vi "VIPropertyPicker.vi"() -> ()   [LabVIEW 2019]
uses:
  VIPropertyPicker/VIPropertyPicker.lvlib
  lib/UI/TreeControl/TreeControlLib.lvlib
  ae6c83ba-cc00-42a4-a275-f8b2c398fdcb.vi
panel:
  out "Last Selection":string
  out "UserMenuNames":string[](array[string])
  out "UserMenuTags":string[](array[string])
  in  "Reload1":bool caption="Reload (CTRL+R)"
  in  "VI Properties":string[](tree)
  in  "Reload2":bool caption="Reload (Ctrl+R)"
  in  "VI List":string(tree)
  in  "Script":string
  in  "Append to Editor in ScriptManager":bool
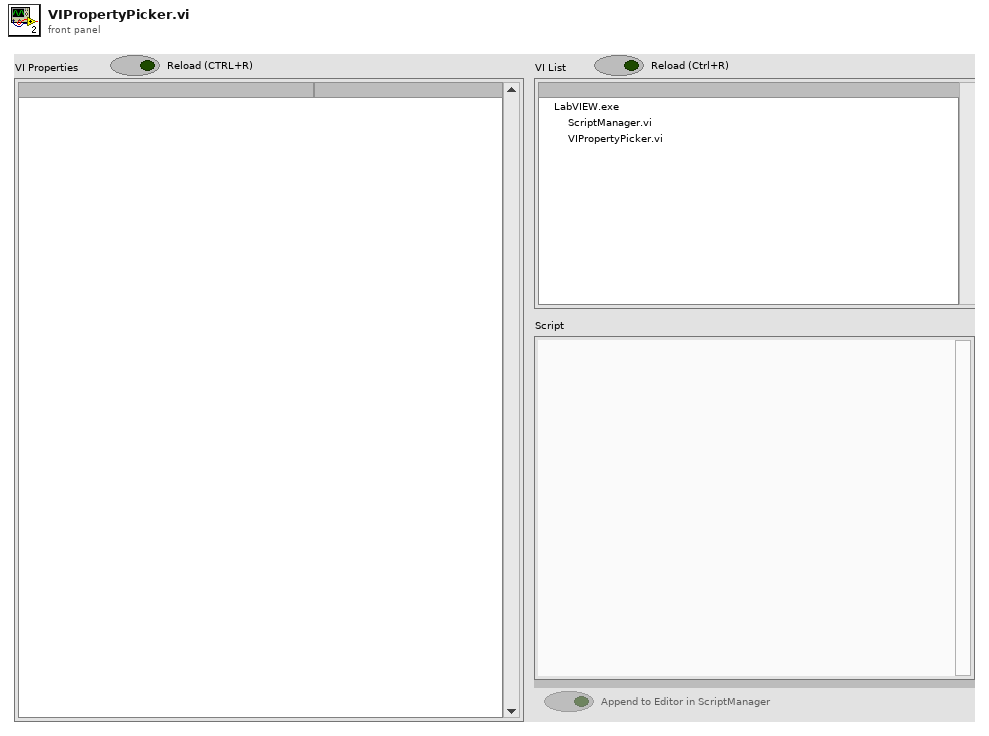
[diagram p1: front panel]
types:
  T1 = enum8{"Enabled", "Disabled", "Disabled and Grayed Out"}
  T2 = cluster{"Name":string, "Include Shift Key?":bool, "Include Ctrl Key?":bool, "Shortcut Key":string}[]
  T3 = cluster{"Closed Nodes":string[], "Selection":string[], "Defer Panel Update":bool, "FocusItem":string}
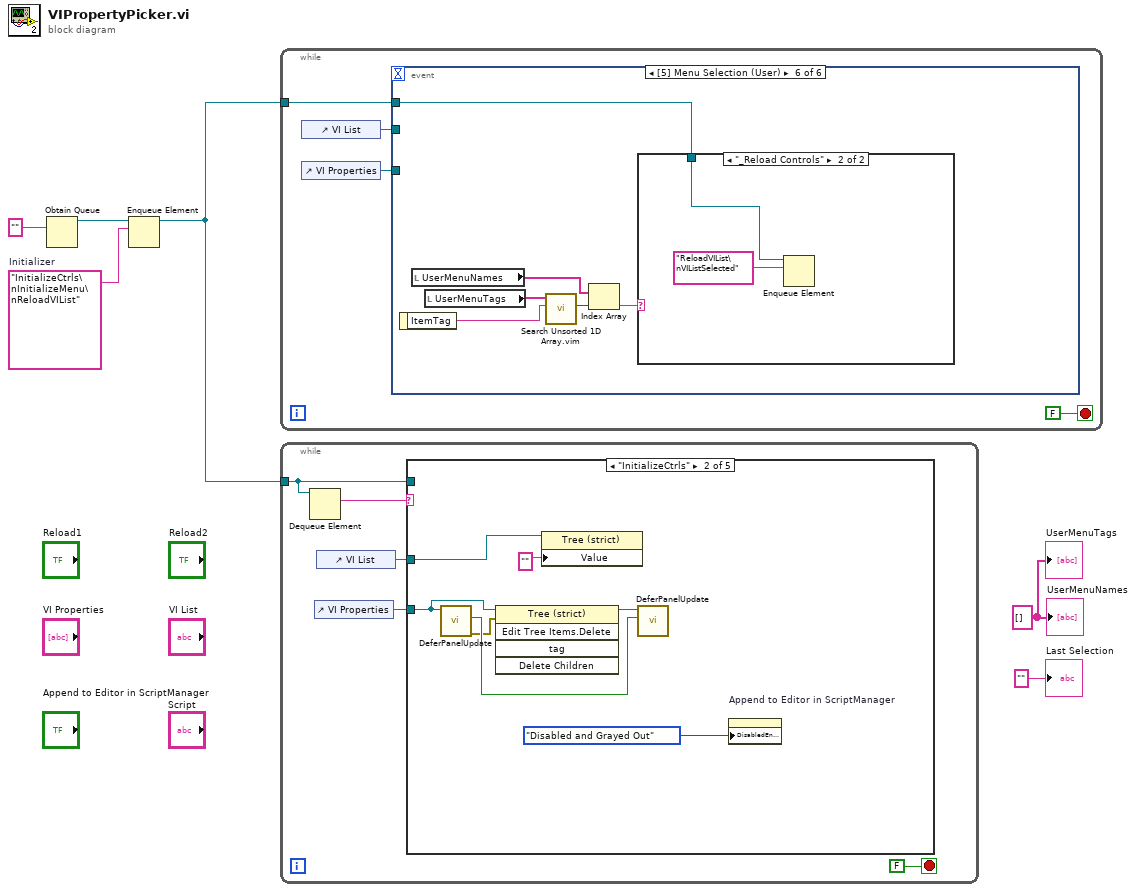
[diagram p0: block diagram]
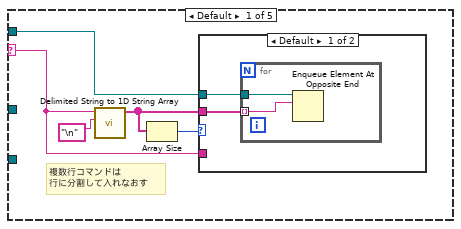
[diagram p2: hidden frame]
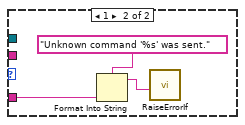
[diagram p3: hidden frame]
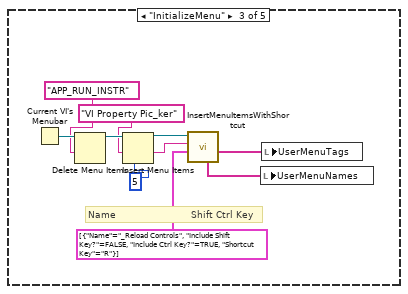
[diagram p4: hidden frame]
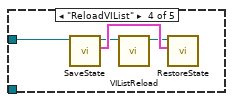
[diagram p5: hidden frame]
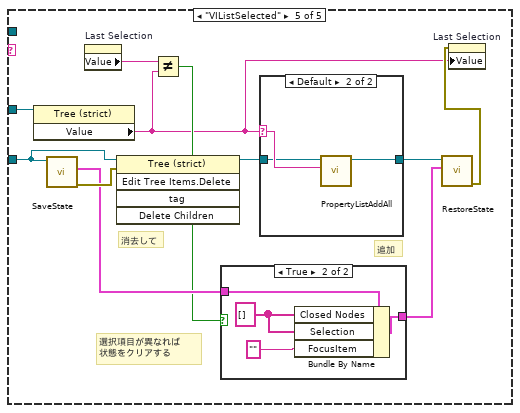
[diagram p6: hidden frame]
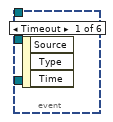
[diagram p9: hidden frame]
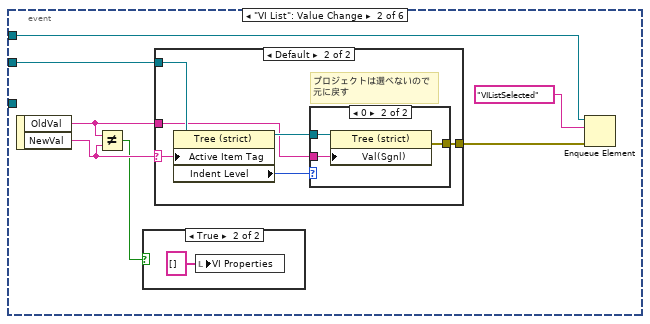
[diagram p10: hidden frame]
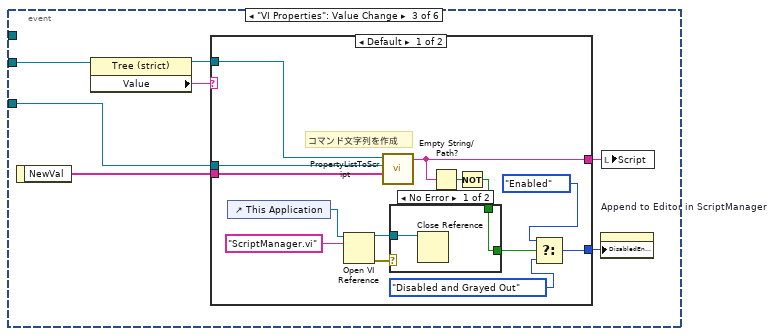
[diagram p14: hidden frame]
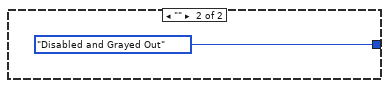
[diagram p16: hidden frame]
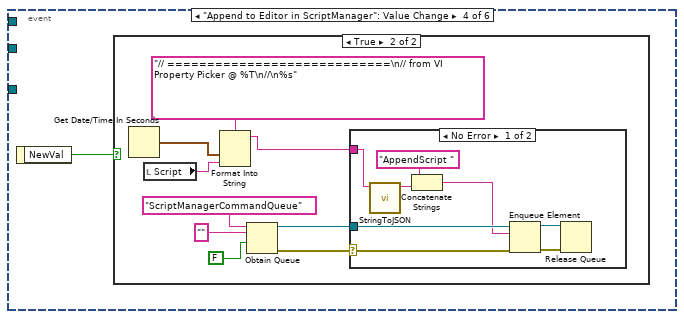
[diagram p17: hidden frame]
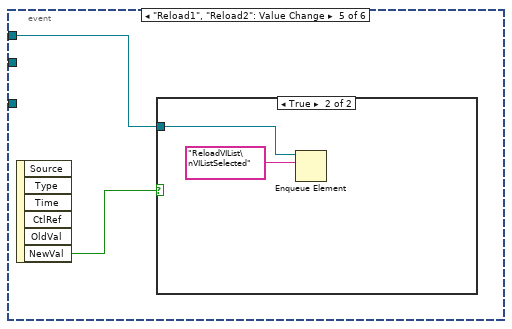
[diagram p20: hidden frame]
diagram:
  w1 = string[] [] ("UserMenuNames")
  w3 = "InitializeCtrls\nInitializeMenu\nReloadVIList"  # Initializer
  n1 = Obtain Queue(element data type="") -> (queue out=w5:refnum<queue>)  [unwired: 4 in, 2 out]
  n2 = Enqueue Element(queue=w5, element=w3) -> (queue out=w4:refnum<queue>)  [unwired: 2 in, 2 out]
  n3 = while {
    tunnel: w4 -> [w9]
    stop <- FALSE stop-if-true
    n4 = control-ref of="VI List"() -> (w8:refnum<vi>)
    n5 = control-ref of="VI Properties"() -> (w7:refnum<vi>)
    n6 = event shown="[5] Menu Selection (User)" {
      selector: _ -> [_ _ _ _ _ _]
      dyn-events: _ -> [_ _ _ _ _ _]
      timeout: _ -> [_ _ _ _ _ _]
      tunnel: w9 -> [_ w16 _ _ w70 w74]
      tunnel: w8 -> [_ w17 w31 _ _ _]
      tunnel: w7 -> [_ _ w33 _ _ _]
      event Timeout {
        n7 = event-data() -> ()  [unwired: 1 in, 3 out]
      }
      event "VI List": Value Change {
        n8 = event-data() -> ("OldVal"=w13:string, "NewVal"=w12:string)  [unwired: 1 in]
        n9 = Not Equal?(x=w13, y=w12) -> (x != y?=w11:bool)
        n10 = case shown="True" w11 {
          frame False {
          }
          frame True {
            n11 = local write "VI Properties"(string[] [] ("VI Properties")) -> ()
          }
        }
        n12 = case shown="Default" w12 {
          selector: w12 -> [_ w19]
          tunnel: w17 -> [_ w24]
          tunnel: [_ w21] -> w14
          tunnel: w13 -> [_ w20]
          frame "" {
          }
          frame Default {
            # "プロジェクトは選べないので\n元に戻す"
            n13 = property class="Tree (strict)"(reference=w24, "Active Item Tag"=w19) -> (reference out=w23:refnum<vi>, "Indent Level"=w22:i32)  [unwired: 1 in, 1 out]
            n14 = case shown="0" w22 {
              tunnel: w23 -> [_ w27]
              tunnel: w20 -> [_ w26]
              tunnel: [_ w25] -> w21
              frame Default {
              }
              frame 0 {
                n15 = property class="Tree (strict)"(reference=w27, "Val(Sgnl)"=w26) -> (error out=w25:errorcluster)  [unwired: 1 in, 1 out]
              }
            }
          }
        }
        n16 = Enqueue Element(queue=w16, element="VIListSelected", error in (no error)=w14) -> ()  [unwired: 1 in, 3 out]
      }
      event "VI Properties": Value Change {
        n17 = event-data() -> ("NewVal"=w34:string[])  [unwired: 1 in]
        n18 = property class="Tree (strict)"(reference=w31) -> (reference out=w29:refnum<vi>, "Value"=w30:string)  [unwired: 1 in, 1 out]
        n19 = case shown="Default" w30 {
          tunnel: w34 -> [w48 _]
          tunnel: w33 -> [w47 _]
          tunnel: [w42 _] -> w32
          tunnel: w29 -> [w35 _]
          tunnel: [w36 T1."Disabled and Grayed Out" ("Disabled")] -> w28
          frame Default {
            # "コマンド文字列を作成"
            n20 = control-ref of="This Application"() -> (w46:refnum<vi>)
            n21 = Open VI Reference(application reference (local)=w46, vi path="ScriptManager.vi") -> (vi reference=w44:refnum<vi>, error out=w43:errorcluster)  [unwired: 4 in]
            n22 = call "PropertyListToScript.vi"("NewVal"=w48, "VI Properties"=w47, "TreeControl in"=w35) -> ("Script"=w42:string)  [unwired: 8 in]
            n23 = Empty String/Path?(string/path=w42) -> (empty?=w41:bool)
            n24 = Not(x=w41) -> (.not. x?=w39:bool)
            n25 = case shown="No Error" w43 {
              tunnel: w44 -> [w50 _]
              tunnel: [w49 _] -> w38
              tunnel: w39 -> [w49 _]
              frame No Error {
                n26 = Close Reference(reference=w50) -> ()  [unwired: 1 in, 1 out]
              }
              frame Error {
              }
            }
            n27 = Select(t=T1."Enabled" ("Disabled"), s=w38, f=T1."Disabled and Grayed Out" ("Disabled")) -> (s? t:f=w36:T1)
          }
          frame "" {
          }
        }
        n28 = property on="Append to Editor in ScriptManager" class="Bool (strict)"("DisabledEnum"=w28) -> ()  [unwired: 2 in, 2 out]
        n29 = local write "Script"(w32) -> ()
      }
      event "Append to Editor in ScriptManager": Value Change {
        n30 = event-data() -> ("NewVal"=w52:bool)  [unwired: 1 in]
        n31 = case shown="True" w52 {
          frame False {
          }
          frame True {
            n32 = Get Date/Time In Seconds() -> (seconds since 1Jan1904=w53:timestamp)
            n33 = local read "Script"() -> (w54:string)
            n34 = Format Into String(format string="// ============================\n// from VI Property Picker @ %T\n//\n%s", w53, w54) -> (resulting string=w56:string)  [unwired: 2 in, 1 out]
            n35 = Obtain Queue(name (unnamed)="ScriptManagerCommandQueue", element data type="", create if not found? (T)=FALSE) -> (queue out=w58:refnum<queue>, error out=w57:errorcluster)  [unwired: 2 in, 1 out]
            n36 = case shown="No Error" w57 {
              selector: w57 -> [w62 _]
              tunnel: w56 -> [w69 _]
              tunnel: w58 -> [w67 _]
              frame No Error {
                n37 = call "StringToJSON.vi"("input text"=w69) -> ("JSON string"=w68:string)  [unwired: 10 in]
                n38 = Concatenate Strings("AppendScript " ("string"), w68) -> (w64:string)
                n39 = Enqueue Element(queue=w67, element=w64, error in (no error)=w62) -> (queue out=w66:refnum<queue>, error out=w65:errorcluster)  [unwired: 1 in, 1 out]
                n40 = Release Queue(queue=w66, error in (no error)=w65) -> ()  [unwired: 1 in, 3 out]
              }
              frame Error {
              }
            }
          }
        }
      }
      event "Reload1", "Reload2": Value Change {
        n41 = event-data() -> ("NewVal"=w71:bool)  [unwired: 1 in, 5 out]
        n42 = case shown="True" w71 {
          tunnel: w70 -> [_ w73]
          frame False {
          }
          frame True {
            n43 = Enqueue Element(queue=w73, element="ReloadVIList\nVIListSelected") -> ()  [unwired: 2 in, 3 out]
          }
        }
      }
      event Menu Selection (User) {
        n44 = event-data() -> ("ItemTag"=w78:string)  [unwired: 1 in]
        n45 = local read "UserMenuNames"() -> (w77:string[])
        n46 = local read "UserMenuTags"() -> (w79:string[])
        n47 = call "Search Unsorted 1D Array.vim"("element"=w78, "unsorted 1D array"=w79) -> ("index of element"=w76:i32)  [unwired: 9 in]
        n48 = Index Array(array=w77, index=w76) -> (element=w75:string)
        n49 = case shown="\"_Reload Controls\"" w75 {
          selector: w75 -> [w80 _]
          tunnel: w74 -> [_ w83]
          frame Default {
            n50 = Concatenate Strings("Unknown menu item was selected:\n", w80) -> (w82:string)
            n51 = call "RaiseErrorIf.vi"("error message"=w82) -> ()  [unwired: 10 in, 1 out]
          }
          frame "_Reload Controls" {
            n52 = Enqueue Element(queue=w83, element="ReloadVIList\nVIListSelected") -> ()  [unwired: 2 in, 3 out]
          }
        }
      }
    }
  }
  n53 = while {
    tunnel: w4 -> [w86]
    stop <- FALSE stop-if-true
    n54 = Dequeue Element(queue=w86) -> (element=w88:string)  [unwired: 2 in, 3 out]
    n55 = control-ref of="VI Properties"() -> (w85:refnum<vi>)
    n56 = control-ref of="VI List"() -> (w87:refnum<vi>)
    n57 = case shown="\"InitializeCtrls\"" w88 {
      selector: w88 -> [w92 _ _ _ _]
      tunnel: w87 -> [_ w104 _ w119 w133]
      tunnel: w86 -> [w90 _ _ _ _]
      tunnel: w85 -> [_ w106 _ _ w130]
      frame Default {
        # "複数行コマンドは\n行に分割して入れなおす"
        n58 = call <vilib>:"Delimited String to 1D String Array.vi"("delimiter"="\n", "delimited string"=w92) -> ("string array"=w91:string[])  [unwired: 9 in]
        n59 = Array Size(array=w91) -> (size(s)=w93:i32)
        n60 = case shown="Default" w93 {
          tunnel: w92 -> [_ w100]
          tunnel: w91 -> [w96 _]
          tunnel: w90 -> [w95 _]
          frame Default {
            n61 = for {
              tunnel: w96 -> [w97] mode=indexing
              tunnel: w95 -> [w98]
              n62 = Enqueue Element At Opposite End(queue=w98, element=w97) -> ()  [unwired: 2 in, 3 out]
            }
          }
          frame 1 {
            n63 = Format Into String(format string="Unknown command '%s' was sent." ("error message"), w100) -> (resulting string=w99:string)  [unwired: 2 in, 1 out]
            n64 = call "RaiseErrorIf.vi"("error message"=w99) -> ()  [unwired: 10 in, 1 out]
          }
        }
      }
      frame "InitializeCtrls" {
        n65 = call "DeferPanelUpdate.vi"("Control in"=w106) -> ("error out"=w107:errorcluster, "Defer Panel Updates Old"=w108:bool)  [unwired: 8 in, 1 out]
        n66 = invoke class="Tree (strict)" method="Edit Tree Items.Delete"(reference=w106, error in=w107) -> (reference out=w105:refnum<vi>)  [unwired: 3 in, 4 out]
        n67 = property class="Tree (strict)"(reference=w104, "Value"="") -> ()  [unwired: 1 in, 2 out]
        n68 = call "DeferPanelUpdate.vi"("Defer Panel Updates (T)"=w108, "Control in"=w105) -> ()  [unwired: 7 in, 3 out]
        n69 = property on="Append to Editor in ScriptManager" class="Bool (strict)"("DisabledEnum"=T1."Disabled and Grayed Out" ("Disabled")) -> ()  [unwired: 2 in, 2 out]
      }
      frame "InitializeMenu" {
        # "Name                         Shift Ctrl Key"
        n70 = Current VI's Menubar() -> (w115:refnum<k9>)
        n71 = Delete Menu Items(7:"APP_RUN_INSTR", 9:w115) -> (3:w118:refnum<k9>)  [unwired: 2 in, 1 out]
        n72 = Insert Menu Items(4:5, 7:"VI Property Pic_ker", 9:w118) -> (1:w117:string, 3:w116:refnum<k9>)  [unwired: 3 in, 1 out]
        n73 = call "InsertMenuItemsWithShortcut.vi"("Sub Items"=T2 [{"Name"="_Reload Controls", "Include Shift Key?"=FALSE, "Include Ctrl Key?"=TRUE, "Shortcut Key"="R"}] ("Menu Short Cut"), "Target Tag"=w117, "menu ref"=w116) -> ("Sub Item Tags"=w110:string[], "Sub Item Names"=w109:string[])  [unwired: 5 in, 2 out]
        n74 = local write "UserMenuNames"(w109) -> ()
        n75 = local write "UserMenuTags"(w110) -> ()
      }
      frame "ReloadVIList" {
        n76 = call "SaveState.vi"("TreeControl in"=w119) -> ("State"=w122:T3, "TreeControl out"=w120:refnum<vi>)  [unwired: 8 in, 1 out]
        n77 = call "VIListReload.vi"("VI List in"=w120) -> ("VI List out"=w121:refnum<vi>)  [unwired: 10 in]
        n78 = call "RestoreState.vi"("State"=w122, "TreeControl in"=w121) -> ()  [unwired: 8 in, 2 out]
      }
      frame "VIListSelected" {
        # "選択項目が異なれば\n状態をクリアする"
        # "追加"
        # "消去して"
        n79 = property class="Tree (strict)"(reference=w133) -> ("Value"=w123:string)  [unwired: 1 in, 2 out]
        n80 = call "SaveState.vi"("TreeControl in"=w130) -> ("error out"=w129:errorcluster, "State"=w127:T3)  [unwired: 8 in, 1 out]
        n81 = property on="Last Selection" class="Str"() -> ("Value"=w128:string)  [unwired: 2 in, 2 out]
        n82 = invoke class="Tree (strict)" method="Edit Tree Items.Delete"(reference=w130, error in=w129) -> (reference out=w132:refnum<vi>)  [unwired: 3 in, 4 out]
        n83 = Not Equal?(x=w128, y=w123) -> (x != y?=w125:bool)
        n84 = case shown="True" w125 {
          tunnel: w127 -> [w134 w138]
          tunnel: [w134 w137] -> w126
          frame False {
          }
          frame True {
            w136 = string[] [] ("Closed Nodes")
            n85 = Bundle By Name(cluster=w138, "Closed Nodes"=w136, "Selection"=w136, "FocusItem"="") -> (w137:T3)
          }
        }
        n86 = case shown="Default" w123 {
          selector: w123 -> [_ w141]
          tunnel: w132 -> [w139 w140]
          tunnel: [w139 w142] -> w131
          frame "" {
          }
          frame Default {
            n87 = call "PropertyListAddAll.vi"("VITag"=w141, "PropertyList in"=w140) -> ("PropertyList out"=w142:refnum<vi>)  [unwired: 9 in]
          }
        }
        n88 = call "RestoreState.vi"("State"=w126, "TreeControl in"=w131) -> ("error out"=w124:errorcluster)  [unwired: 8 in, 1 out]
        n89 = property on="Last Selection" class="Str"(error in=w124, "Value"=w123) -> ()  [unwired: 1 in, 2 out]
      }
    }
  }
  "UserMenuTags" <- w1
  "UserMenuNames" <- w1
  "Last Selection" <- "" ("Last Selection")
